vi "Anritsu Optical Power Meter (No Objects).vi"(8 "error in":errorcluster, 11 "Cluster In":T13={"Channel Names"=[], "Channel Units"=[], "Most Recent Data Points"=[], "History Buffers"=[], "Ring Buffers"=[], "Averaging"=enum."On", "Units"=enum."Watt", "Measuring rate"=enum."Hold", "Unit Range"=enum."10 mW (+10 dBm)", "Calibration Factor"=-26.67, "Auto Ranging?"=enum."Off"}) -> (0 "error out":errorcluster, 3 "Cluster Out":T13={"Channel Names"=[], "Channel Units"=[], "Most Recent Data Points"=[], "History Buffers"=[], "Ring Buffers"=[], "Averaging"=enum."On", "Units"=enum."Watt", "Measuring rate"=enum."Hold", "Unit Range"=enum."10 mW (+10 dBm)", "Calibration Factor"=-26.67, "Auto Ranging?"=enum."Off"})   [LabVIEW 2009]
uses:
  Utility Classes/Readable/Channel Names.ctl
  Utility Classes/Readable/Channel Units.ctl
  Utility Classes/Readable/Data Points.ctl
  Utility Classes/Readable/Data Point.ctl
  Utility Classes/Readable/Time.ctl
  Utility Classes/Readable/X.ctl
  Utility Classes/Readable/TX Graph.ctl
  Anritsu Power Meter/Public/Averaging control.ctl
  Anritsu Power Meter/Public/Display control.ctl
  Anritsu Power Meter/Public/Measuring rate control.ctl
  Anritsu Power Meter/Public/Range control watts and dBm.ctl
  Anritsu Power Meter/Public/Auto Range control.ctl
  Utility Classes/Readable/Readable.lvclass
panel:
  out "Status":string
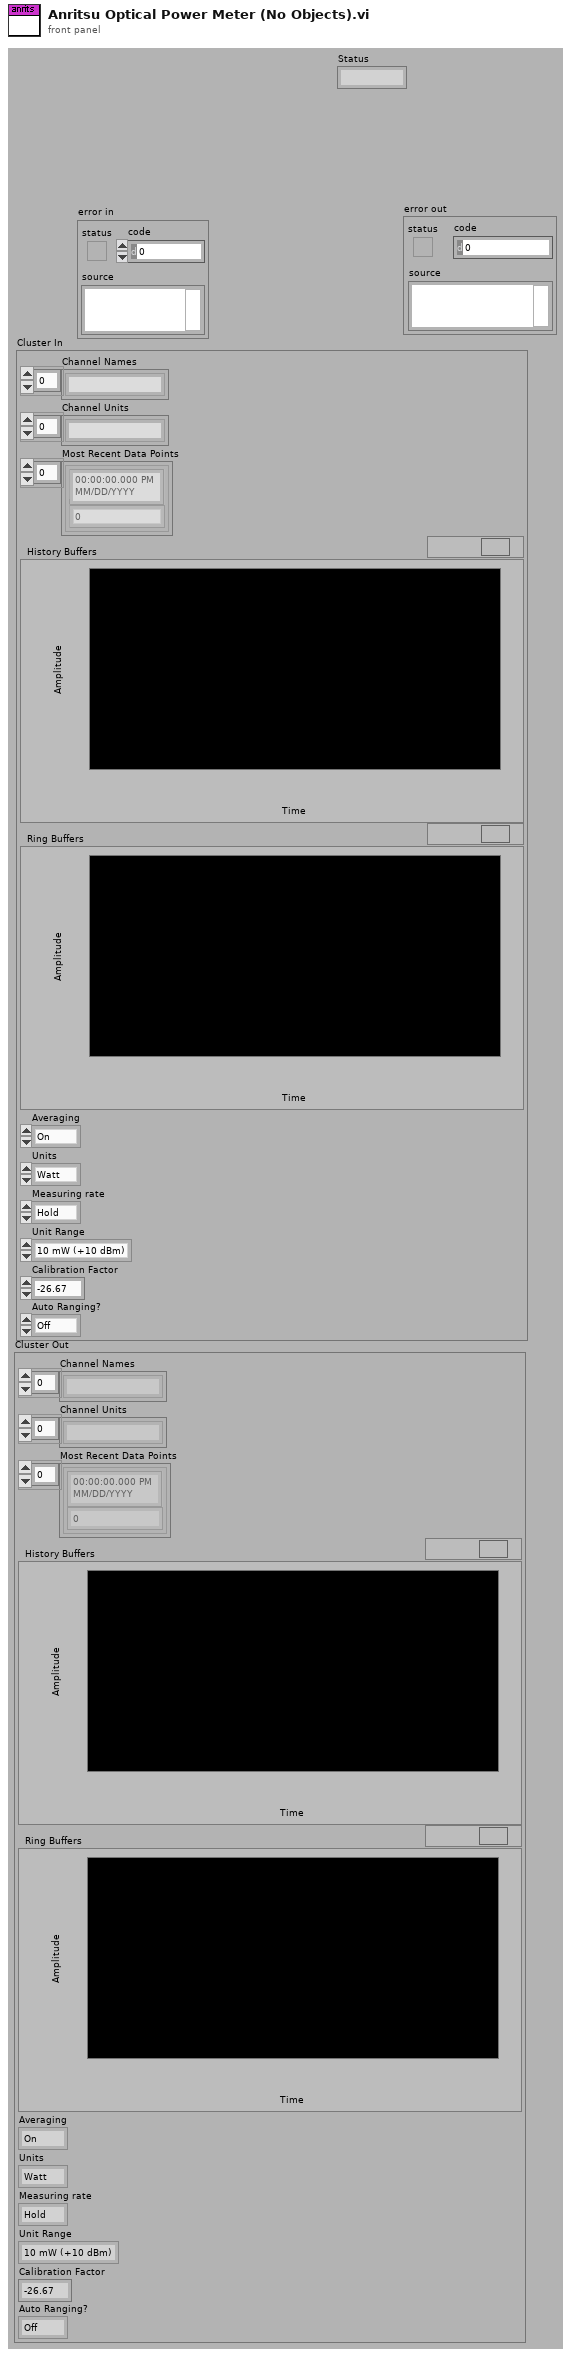
[diagram p1: front panel]
types:
  T1 = typedef "Readable.lvclass/Channel Names.ctl" = string[]
  T2 = typedef "Readable.lvclass/Channel Units.ctl" = string[]
  T3 = typedef "Readable.lvclass/Data Points.ctl" = T4[]
  T4 = typedef "Readable.lvclass/Data Point.ctl" = cluster{"t":T5, "x":T6}
  T5 = typedef "Readable.lvclass/Time.ctl" = timestamp
  T6 = typedef "Readable.lvclass/X.ctl" = dbl
  T7 = typedef "Readable.lvclass/TX Graph.ctl" = cluster{"Data Points":cluster{"t":timestamp, "x":dbl}[]}[]
  T8 = typedef "Averaging control.ctl" = enum16{"On", "Off"}
  T9 = typedef "Display control.ctl" = enum16{"Watt", "dBm", "dB (REL)"}
  T10 = typedef "Measuring rate control.ctl" = enum16{"Hold", "Free Run", "Exit Trigger"}
  T11 = typedef "Range control watts and dBm.ctl" = enum16{"10 mW (+10 dBm)", "1 mW (0 dBm)", "100 uW (-10 dBm)", "10 uW (-20 dBm)", "1 uW (-30 dBm)", "100 nW (-40 dBm)", "10 nW (-50 dBm)", "1 nW (-60 dBm)", "100 pW (-70 dBm)", "10 pW (-80 dBm)"}
  T12 = typedef "Auto Range control.ctl" = enum16{"Off", "On"}
  T13 = cluster{"Channel Names":T1, "Channel Units":T2, "Most Recent Data Points":T3, "History Buffers":T7, "Ring Buffers":T7, "Averaging":T8, "Units":T9, "Measuring rate":T10, "Unit Range":T11, "Calibration Factor":dbl, "Auto Ranging?":T12}
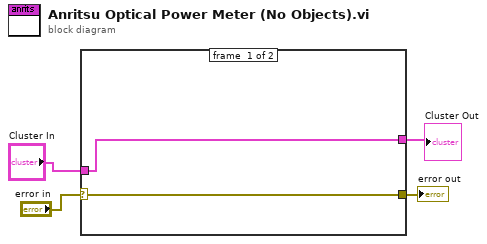
[diagram p0: block diagram]
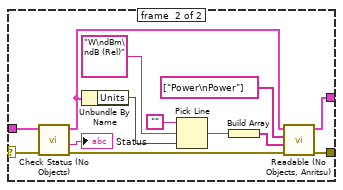
[diagram p2: hidden frame]
diagram:
  n1 = case shown="No Error" "error in" {
    selector: "error in" -> [w6 w9]
    tunnel: [w5 w15] -> w2
    tunnel: [w6 w17] -> w4
    tunnel: "Cluster In" -> [w5 w7]
    frame #0 {
    }
    frame #1 {
      n2 = call "Check Status (No Objects).vi"("error in (no error)"=w9, "Cluster In"=w7) -> ("error out"=w16:errorcluster, "Status"=→"Status":string, "Cluster Out"=w8:T13)  [unwired: 6 in, 1 out]
      n3 = Unbundle By Name(w8) -> ("Units"=w14:T9)
      n4 = Pick Line(string ("")="", multi-line string="W\ndBm\ndB (Rel)" ("string (\"\")"), line index=w14) -> (output string=w13:string)
      n5 = Build Array(w13) -> (w12:string[])
      n6 = call "Readable (No Objects, Anritsu).vi"("error in (no error)"=w16, "Channel Units"=w12, "Channel Names"=T1 ["Power\nPower"], "Cluster In"=w8) -> ("error out"=w17:errorcluster, "Cluster Out"=w15:T13)  [unwired: 6 in]
    }
  }
  "error out" <- w4
  "Cluster Out" <- w2
